vi "CompilerCombinePulseBools.vi"(1 "Raw pulse":T2) -> (0 "Combined pulse":T1)   [LabVIEW 2017]
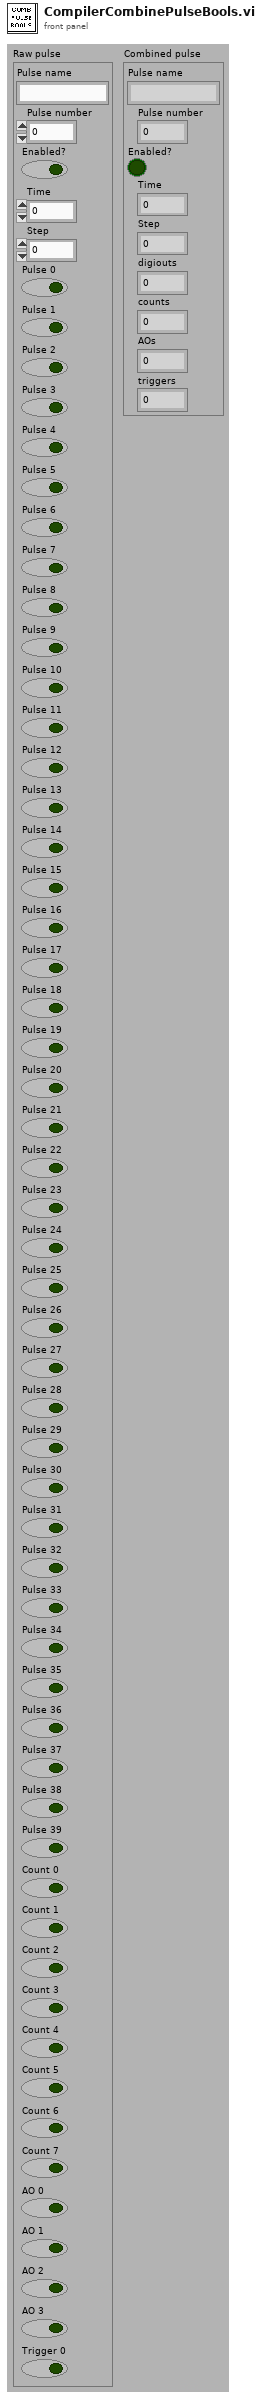
[diagram p1: front panel]
types:
  T1 = cluster{"Pulse name":string, "Pulse number":i32, "Enabled?":bool, "Time":dbl, "Step":dbl, "digiouts":u64, "counts":u8, "AOs":u8, "triggers":u8}
  T2 = cluster{"Pulse name":string, "Pulse number":i32, "Enabled?":bool, "Time":dbl, "Step":dbl, "Pulse 0":bool, "Pulse 1":bool, "Pulse 2":bool, "Pulse 3":bool, "Pulse 4":bool, "Pulse 5":bool, "Pulse 6":bool, "Pulse 7":bool, "Pulse 8":bool, "Pulse 9":bool, "Pulse 10":bool, "Pulse 11":bool, "Pulse 12":bool, "Pulse 13":bool, "Pulse 14":bool, "Pulse 15":bool, "Pulse 16":bool, "Pulse 17":bool, "Pulse 18":bool, "Pulse 19":bool, "Pulse 20":bool, "Pulse 21":bool, "Pulse 22":bool, "Pulse 23":bool, "Pulse 24":bool, "Pulse 25":bool, "Pulse 26":bool, "Pulse 27":bool, "Pulse 28":bool, "Pulse 29":bool, "Pulse 30":bool, "Pulse 31":bool, "Pulse 32":bool, "Pulse 33":bool, "Pulse 34":bool, "Pulse 35":bool, "Pulse 36":bool, "Pulse 37":bool, "Pulse 38":bool, "Pulse 39":bool, "Count 0":bool, "Count 1":bool, "Count 2":bool, "Count 3":bool, "Count 4":bool, "Count 5":bool, "Count 6":bool, "Count 7":bool, "AO 0":bool, "AO 1":bool, "AO 2":bool, "AO 3":bool, "Trigger 0":bool}
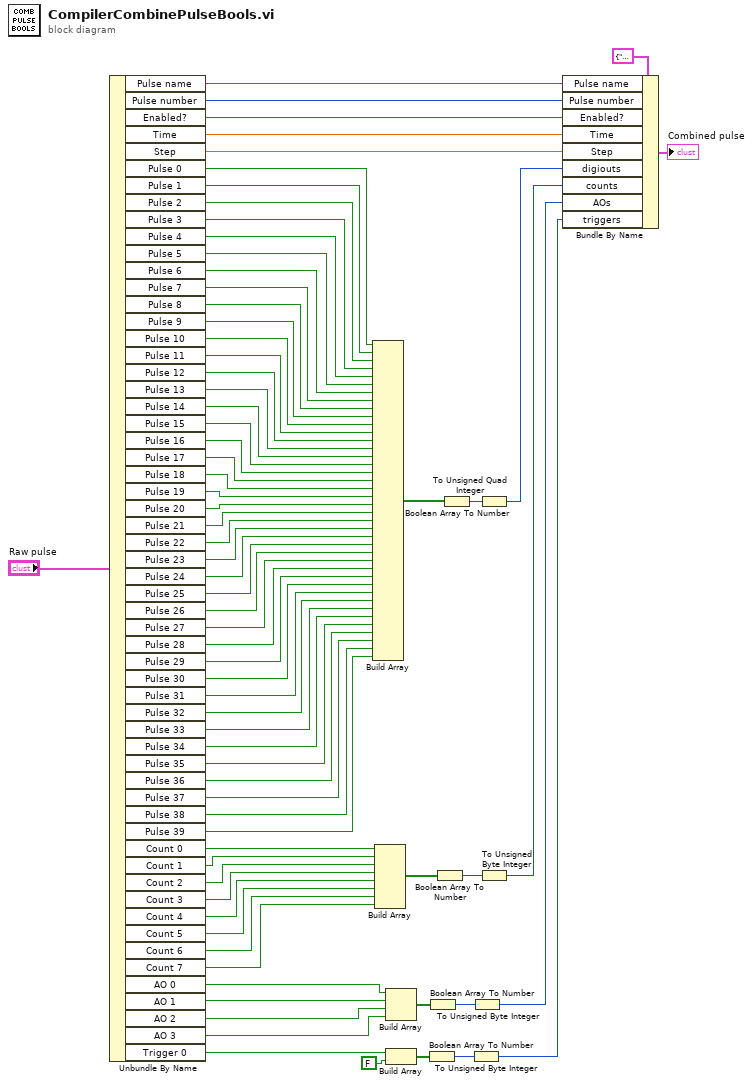
[diagram p0: block diagram]
diagram:
  n1 = Unbundle By Name("Raw pulse") -> ("Pulse name"=w11:string, "Pulse number"=w10:i32, "Enabled?"=w9:bool, "Time"=w8:dbl, "Step"=w7:dbl, "Pulse 0"=w73:bool, "Pulse 1"=w72:bool, "Pulse 2"=w71:bool, "Pulse 3"=w70:bool, "Pulse 4"=w69:bool, "Pulse 5"=w68:bool, "Pulse 6"=w67:bool, "Pulse 7"=w66:bool, "Pulse 8"=w65:bool, "Pulse 9"=w64:bool, "Pulse 10"=w63:bool, "Pulse 11"=w62:bool, "Pulse 12"=w61:bool, "Pulse 13"=w60:bool, "Pulse 14"=w59:bool, "Pulse 15"=w58:bool, "Pulse 16"=w57:bool, "Pulse 17"=w56:bool, "Pulse 18"=w55:bool, "Pulse 19"=w54:bool, "Pulse 20"=w53:bool, "Pulse 21"=w50:bool, "Pulse 22"=w52:bool, "Pulse 23"=w51:bool, "Pulse 24"=w49:bool, "Pulse 25"=w48:bool, "Pulse 26"=w47:bool, "Pulse 27"=w46:bool, "Pulse 28"=w45:bool, "Pulse 29"=w44:bool, "Pulse 30"=w43:bool, "Pulse 31"=w42:bool, "Pulse 32"=w41:bool, "Pulse 33"=w40:bool, "Pulse 34"=w39:bool, "Pulse 35"=w38:bool, "Pulse 36"=w37:bool, "Pulse 37"=w36:bool, "Pulse 38"=w35:bool, "Pulse 39"=w34:bool, "Count 0"=w32:bool, "Count 1"=w31:bool, "Count 2"=w30:bool, "Count 3"=w29:bool, "Count 4"=w28:bool, "Count 5"=w27:bool, "Count 6"=w26:bool, "Count 7"=w25:bool, "AO 0"=w19:bool, "AO 1"=w18:bool, "AO 2"=w17:bool, "AO 3"=w16:bool, "Trigger 0"=w15:bool)
  n2 = Build Array(w73, w72, w71, w70, w69, w68, w67, w66, w65, w64, w63, w62, w61, w60, w59, w58, w57, w56, w55, w54, w53, w50, w52, w51, w49, w48, w47, w46, w45, w44, w43, w42, w41, w40, w39, w38, w37, w36, w35, w34) -> (w33:bool[])
  n3 = Build Array(w32, w31, w30, w29, w28, w27, w26, w25) -> (w13:bool[])
  n4 = Build Array(w19, w18, w17, w16) -> (w20:bool[])
  n5 = Build Array(w15, FALSE ("element")) -> (w23:bool[])
  n6 = Boolean Array To Number(Boolean array=w23) -> (number=w24:u32)
  n7 = Boolean Array To Number(Boolean array=w20) -> (number=w21:u32)
  n8 = Boolean Array To Number(Boolean array=w13) -> (number=w14:u32)
  n9 = Boolean Array To Number(Boolean array=w33) -> (number=w12:u64)
  n10 = To Unsigned Byte Integer(number=w24) -> (unsigned 8bit integer=w3:u8)
  n11 = To Unsigned Byte Integer(number=w21) -> (unsigned 8bit integer=w4:u8)
  n12 = To Unsigned Quad Integer(1:w12) -> (0:w6:u64)
  n13 = To Unsigned Byte Integer(number=w14) -> (unsigned 8bit integer=w5:u8)
  n14 = Bundle By Name(cluster=T1 {"Pulse name"="", "Pulse number"=0, "Enabled?"=FALSE, "Time"=0.0, "Step"=0.0, "digiouts"=0, "counts"=0, "AOs"=0, "triggers"=0} ("output cluster"), "Pulse name"=w11, "Pulse number"=w10, "Enabled?"=w9, "Time"=w8, "Step"=w7, "digiouts"=w6, "counts"=w5, "AOs"=w4, "triggers"=w3) -> (→"Combined pulse":T1)
